vi "Get Switch node.vi"(8 "error in (no error)":errorcluster, 10 "Engine":string="Switch", 11 "ACIR Instrument":refnum<class "ACIR Instrument.lvclass">) -> (0 "error out":errorcluster, 2 "Switch node":refnum<data-value>, 3 "ACIR Instrument out":refnum<class "ACIR Instrument.lvclass">)   [LabVIEW 2025, in "ACIR.lvlib" / "ACIR Instrument.lvclass"]
uses:
  ACIR Instrument.lvclass
  ACIR Instrument.lvclass/ACIR Instrument.ctl
  Users/Public/Documents/Sandia National Labs/TSS Plugin/Abstract Engine.lvlibp/Abstract Instrument/Abstract Instrument.lvclass
  SwitchACIR Channel/SwitchACIR Channel.lvclass
  SwitchACIR Channel configuration/SwitchACIR Channel configuration.lvclass
  Users/Public/Documents/Sandia National Labs/TSS Plugin/CEF.lvlibp/Node/CEF_Node.lvclass
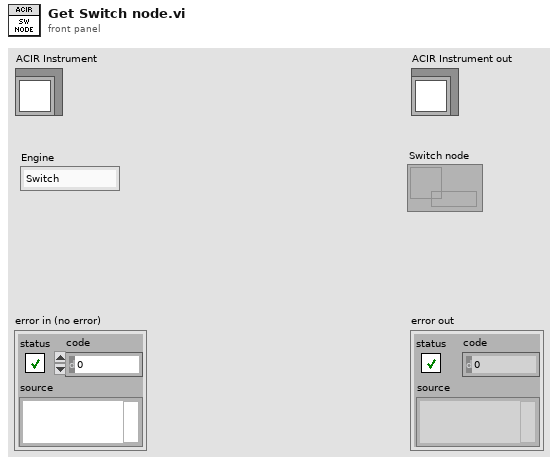
[diagram p1: front panel]
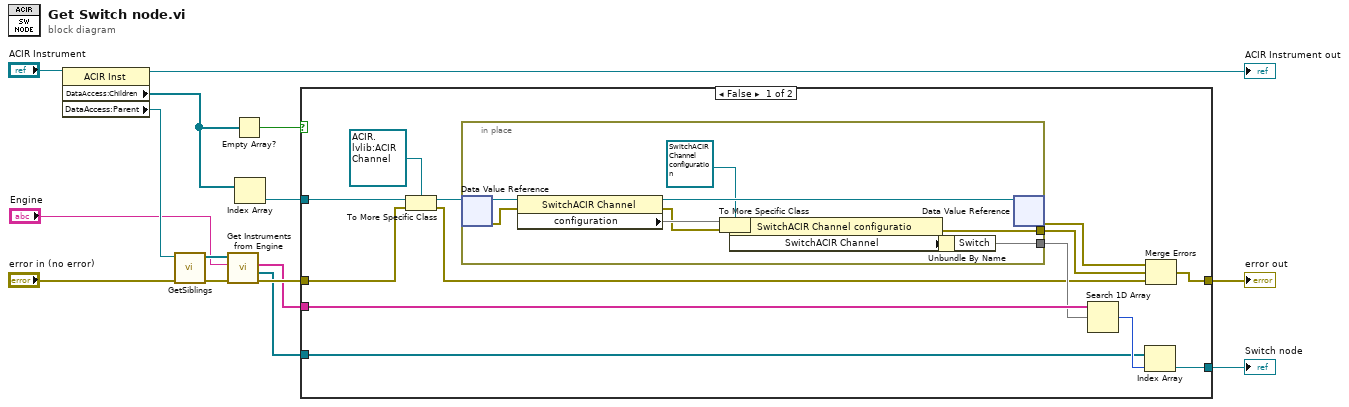
[diagram p0: block diagram]
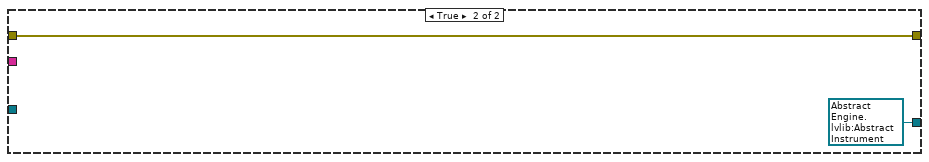
[diagram p2: hidden frame]
diagram:
  n1 = property class="ACIR Inst"(reference="ACIR Instrument") -> (reference out=→"ACIR Instrument out":refnum<class "ACIR Instrument.lvclass">, "DataAccess:Children"=w14:refnum<data-value>[], "DataAccess:Parent"=w3:refnum<data-value>)  [unwired: 1 in, 1 out]
  n2 = call "GetSiblings.vi"("error in"="error in (no error)", "node in"=w3) -> ("error out"=w4:errorcluster, "siblings"=w2:refnum<data-value>[])  [unwired: 8 in]
  n3 = call "Get Instruments from Engine.vi"("error in"=w4, "Engine"="Engine", "Engines"=w2) -> ("error out"=w9:errorcluster, "Instrument nodes"=w6:refnum<data-value>[], "Instruments"=w5:string[])  [unwired: 6 in]
  n4 = Empty Array?(array=w14) -> (empty?=w13:bool)
  n5 = Index Array(array=w14) -> (element=w11:refnum<data-value>)  [unwired: 1 in]
  n6 = case shown="False" w13 {
    tunnel: w5 -> [w25 _]
    tunnel: w6 -> [w23 _]
    tunnel: [w22 refnum<data-value> refnum ("target class")] -> w12
    tunnel: w9 -> [w20 w40]
    tunnel: w11 -> [w21 _]
    tunnel: [w17 w40] -> w10
    frame False {
      n7 = To More Specific Class(target class=refnum<data-value> refnum, reference=w21, error in=w20) -> (specific class reference=w27:refnum<data-value>, error out=w19:errorcluster)
      n8 = in-place {
        in-place-border: [w35] -> w24
        in-place-border: [w30] -> w18
        n9 = in-place-dvr #1(w27) -> (w39:refnum<class "SwitchACIR Channel.lvclass">, w33:errorcluster)
        n10 = property class="SwitchACIR Channel"(reference=w39, error in=w33) -> (reference out=w38:refnum<class "SwitchACIR Channel.lvclass">, error out=w32:errorcluster, "configuration"=w37)
        n11 = To More Specific Class(target class=refnum<class "SwitchACIR Channel configuration.lvclass"> refnum ("ACIR.lvlib:SwitchACIR Channel"), reference=w37, error in=w32) -> (specific class reference=w36:refnum<class "SwitchACIR Channel configuration.lvclass">, error out=w31:errorcluster)
        n12 = property class="SwitchACIR Channel configuratio"(reference=w36, error in=w31) -> (error out=w30:errorcluster, "SwitchACIR Channel"=w34)  [unwired: 1 out]
        n13 = Unbundle By Name(w34) -> ("Switch"=w35)
        n14 = in-place-dvr #1(w38) -> (w16:errorcluster)  [unwired: 1 out]
      }
      n15 = Search 1D Array(1D array=w25, element=w24) -> (index of element=w26:i32)  [unwired: 1 in]
      n16 = Index Array(array=w23, index=w26) -> (element=w22:refnum<data-value>)
      n17 = Merge Errors(w16, w18, w19) -> (w17:errorcluster)
    }
    frame True {
    }
  }
  "error out" <- w10
  "Switch node" <- w12
